vi "get index definition.vi"(10 "channel classification":T1, 11 "ScaleAndLimitModule configuration in":refnum<class "ScaleAndLimitModule configuration.lvclass">) -> (1 "valid?":bool, 2 "index cluster":variant, 3 "ScaleAndLimitModule configuration out":refnum<class "ScaleAndLimitModule configuration.lvclass">)   [LabVIEW 2017, in "ScaleAndLimitModule configuration.lvclass"]
uses:
  ScaleAndLimitModule configuration.lvclass
  <vilib>/NI/Tag Bus Module Framework/channel/channel classification.ctl
  input data indices.ctl
  output data indices.ctl
  parameter data indices.ctl
  result data indices.ctl
  <vilib>/NI/Tag Bus Module Framework/channel/TBM channel.lvclass
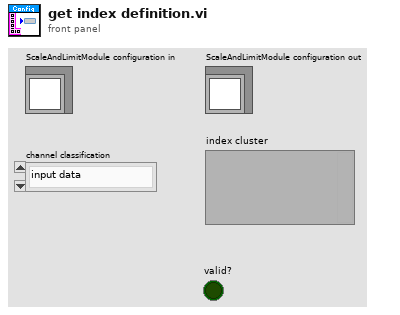
[diagram p1: front panel]
types:
  T1 = typedef "TBM channel.lvclass/channel classification.ctl" = enum16{"input data", "output data", "processing parameter", "processing result"}
  T2 = typedef "ScaleAndLimitModule configuration.lvclass/input data indices.ctl" = cluster{"Boolean.LimitsFlag":i32, "U16.HighLimits":i32, "U16.LowLimits":i32, "String.LimitsString":i32}
  T3 = typedef "ScaleAndLimitModule configuration.lvclass/output data indices.ctl" = cluster{"Boolean.ClearLimits":i32}
  T4 = typedef "ScaleAndLimitModule configuration.lvclass/parameter data indices.ctl" = cluster{"fmwk_placeholder":i32}
  T5 = typedef "ScaleAndLimitModule configuration.lvclass/result data indices.ctl" = cluster{"fmwk_placeholder":i32}
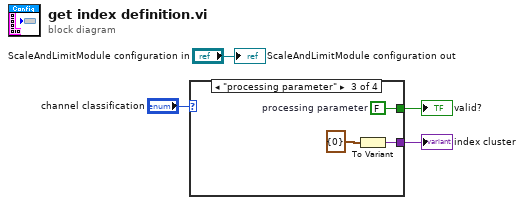
[diagram p0: block diagram]
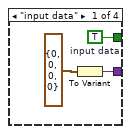
[diagram p2: hidden frame]
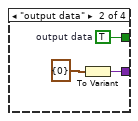
[diagram p3: hidden frame]
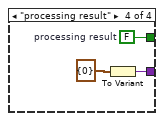
[diagram p4: hidden frame]
diagram:
  n1 = case shown="\"processing parameter\"" "channel classification" {
    tunnel: [w6 w10 w13 w16] -> w2
    tunnel: [w5 w9 w12 w15] -> w1
    frame "input data" {
      w5 = TRUE  # input data
      n2 = To Variant(anything=T2 {"Boolean.LimitsFlag"=0, "U16.HighLimits"=0, "U16.LowLimits"=0, "String.LimitsString"=0} ("Cluster")) -> (Variant=w6:variant)
    }
    frame "output data" {
      w9 = TRUE  # output data
      n3 = To Variant(anything=T3 {"Boolean.ClearLimits"=0} ("Cluster")) -> (Variant=w10:variant)
    }
    frame "processing parameter" {
      w12 = FALSE  # processing parameter
      n4 = To Variant(anything=T4 {"fmwk_placeholder"=0} ("Cluster")) -> (Variant=w13:variant)
    }
    frame "processing result" {
      w15 = FALSE  # processing result
      n5 = To Variant(anything=T5 {"fmwk_placeholder"=0} ("Cluster")) -> (Variant=w16:variant)
    }
  }
  "index cluster" <- w2
  "valid?" <- w1
  "ScaleAndLimitModule configuration out" <- "ScaleAndLimitModule configuration in"
